vi "Read Storage Settings.vi"(8 "error in (no error)":errorcluster, 11 "Controller in":refnum<class "Controller.lvclass">) -> (0 "error out":errorcluster, 2 "Storage Settings":T1, 3 "Controller out":refnum<class "Controller.lvclass">)   [LabVIEW 2021, in "Controller.lvlib" / "Controller.lvclass"]
uses:
  Controller.lvclass
  Typedefs/Image Formats.ctl
  Typedefs/Storage Settings.ctl
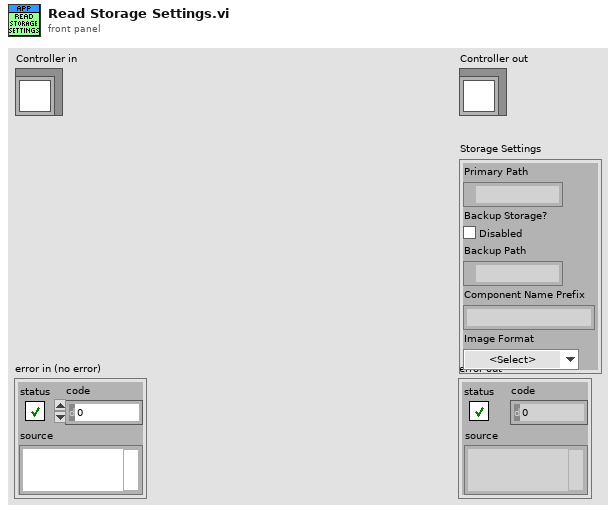
[diagram p1: front panel]
types:
  T1 = typedef "Storage Settings.ctl" = cluster{"Primary Path":path, "Backup Storage?":bool, "Backup Path":path, "Component Name Prefix":string, "Image Format":T2}
  T2 = typedef "Image Formats.ctl" = enum16{"<Select>", "TIFF", "RAW"}
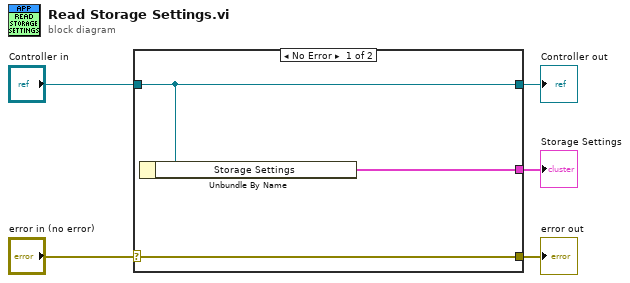
[diagram p0: block diagram]
diagram:
  n1 = case shown="No Error" "error in (no error)" {
    selector: "error in (no error)" -> [w8 w9]
    tunnel: [w8 w9] -> w4
    tunnel: [w7 w10] -> w2
    tunnel: "Controller in" -> [w7 w10]
    tunnel: [w6 _] -> w1
    frame No Error {
      n2 = Unbundle By Name(w7) -> ("Storage Settings"=w6:T1)
    }
    frame Error {
    }
  }
  "error out" <- w4
  "Controller out" <- w2
  "Storage Settings" <- w1
